vi "BarcodeScannerCodeforVideo.vi"() -> ()   [LabVIEW 2016]
uses:
  <vilib>/NXT/Block Support/NXT_InputPort.ctl
  <vilib>/NXT/Block Support/NXT_OutputPort.ctl
  <vilib>/NXT/Dual Mode Library/Sensors/Touch_Count.vi
  <vilib>/NXT/NXTIO Xnodes/NXTIONodeSubVIs/NXTMotorRunDistance.vi
  <vilib>/NXT/Dual Mode Library/Sensors/EV3_Color_Reflect.vi
  <vilib>/NXT/NXTIO Xnodes/NXTIONodeSubVIs/NXTStopMotors.vi
  <vilib>/NXT/Dual Mode Library/Sensors/EV3_Touch_Reset.vi
  <vilib>/NXT/NXTIO Xnodes/AddressXNode/NXTIOAddress.xnode
  <vilib>/NXT/NXTIO Xnodes/NXTIOXNode/NXTIO.xnode
  <vilib>/NXT/Subs/LVHSConnector.ctl
  <vilib>/NXT/LegoClasses/BrickReference/BrickReference.lvclass
panel:
  out "Marble Type 2 Code":i32[](array[numeric])
  out "Marble Count 2 Code":i32[](array[numeric])
  out "Marble Type 4":string
  out "Type 1 count 4":string
  out "Type 2 Count 4":string
  out "Marble Type 4 Code":i32[](array[numeric])
  out "Marble Count 4 Code":i32[](array[numeric])
  out "Marble Type 3":string
  out "Type 2 Count 3":string
  out "Type 1 Count 3":string
  out "Marble Count 3":i32[](array[numeric])
  out "Marble Type 3":i32[](array[numeric])
  out "Marble Type 2":string
  out "Type 2 Count 2":string
  out "Type 1 Count 2":string
  out "Marble Type code":i32[](array[numeric])
  out "Marble Size code":i32[](array[numeric])
  out "Marble Type":string
  out "Type 2 Count":string
  out "Type 1 Count":string
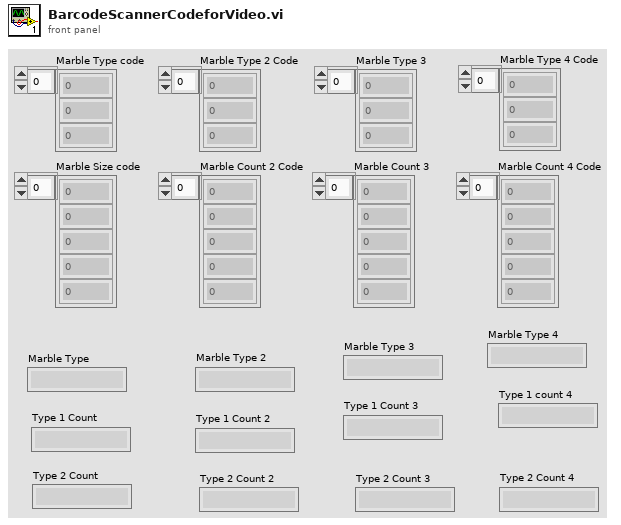
[diagram p1: front panel]
types:
  T1 = typedef "NXT_InputPort.ctl" = u32
  T2 = typedef "LVHSConnector.ctl" = refnum<class "BrickReference.lvclass">
  T3 = typedef "NXT_OutputPort.ctl" = u8
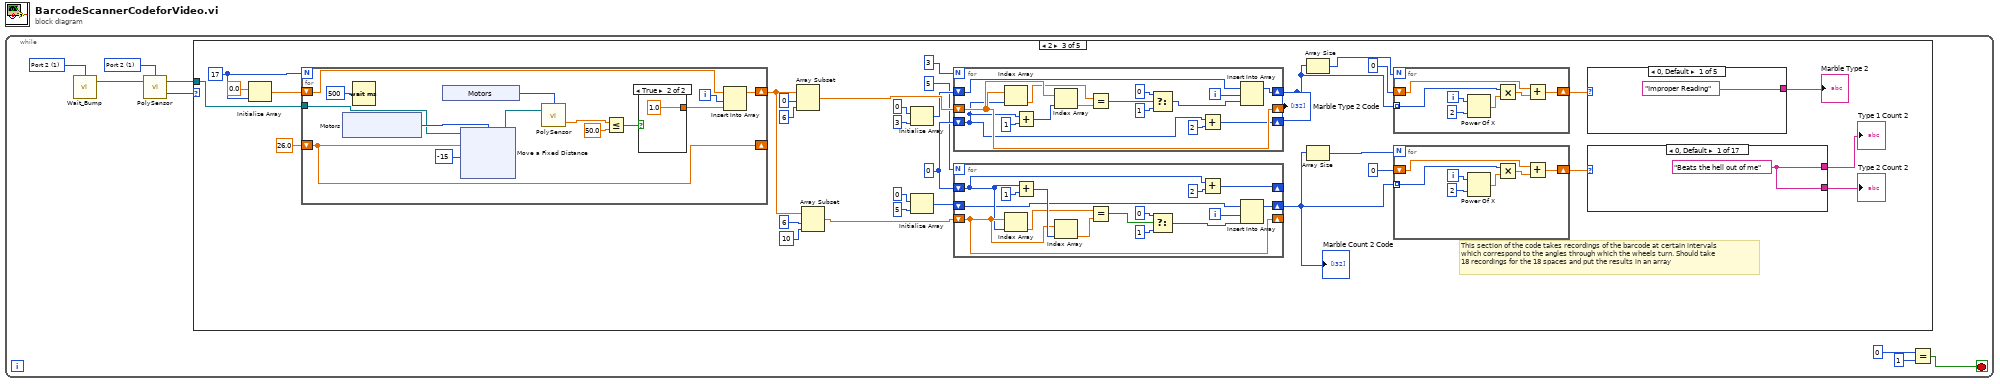
[diagram p0: block diagram]
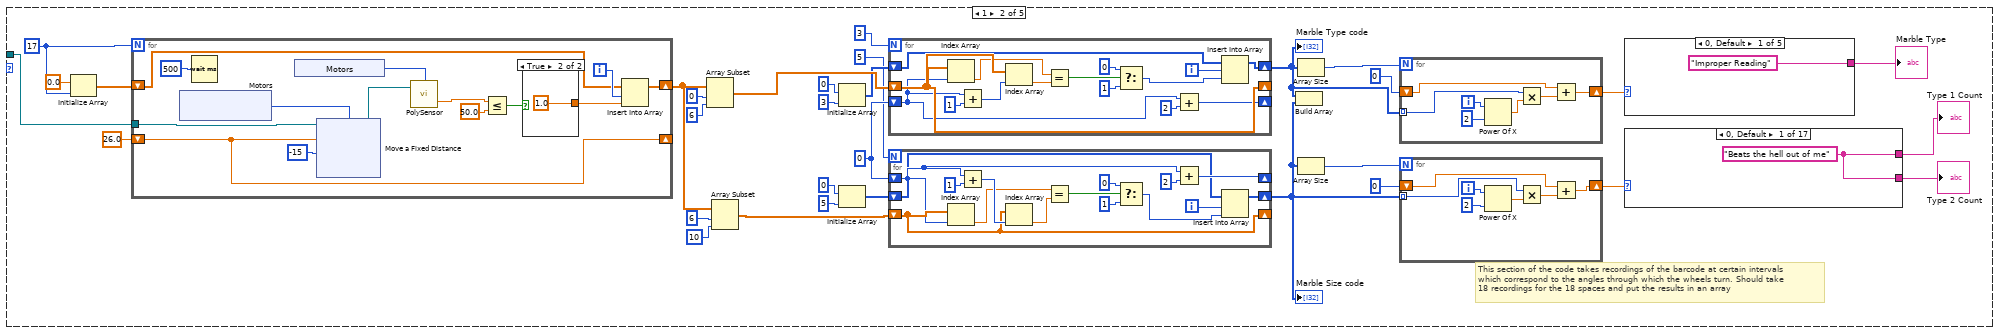
[diagram p3: hidden frame]
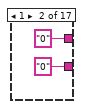
[diagram p4: hidden frame]
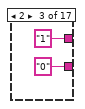
[diagram p5: hidden frame]
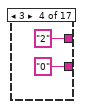
[diagram p6: hidden frame]
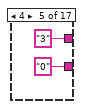
[diagram p7: hidden frame]
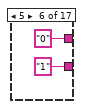
[diagram p8: hidden frame]
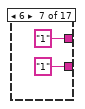
[diagram p9: hidden frame]
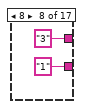
[diagram p10: hidden frame]
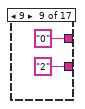
[diagram p11: hidden frame]
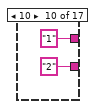
[diagram p12: hidden frame]
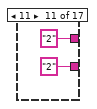
[diagram p13: hidden frame]
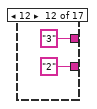
[diagram p14: hidden frame]
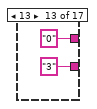
[diagram p15: hidden frame]
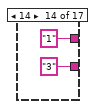
[diagram p16: hidden frame]
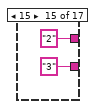
[diagram p17: hidden frame]
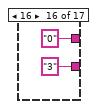
[diagram p18: hidden frame]
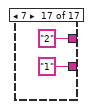
[diagram p19: hidden frame]
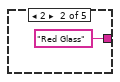
[diagram p20: hidden frame]
diagram:
  n1 = while {
    stop <- w1 stop-if-true
    w4 = T1 1 items=["Port 1", "Port 2", "Port 3", "Port 4"] ("Port (Port 1)")
    w5 = T1 1 items=["Port 1", "Port 2", "Port 3", "Port 4"] ("Port (Port 1)")
    n2 = call <vilib>:"Wait_Bump.vi"("Port (Port 1)"=w5) -> ("NXT/EV3"=w7:T2)  [unwired: 3 in]
    n3 = call-poly <vilib>:"PolySensor.vi"("NXT/EV3"=w7, "Port (Port 1)"=w4) -> ("Count"=w8:i16, "NXT/EV3"=w6:T2)  [unwired: 1 in]
    n4 = case shown="2" w8 {
      tunnel: w6 -> [_ w9 w151 w293 w444]
      frame 0, Default {
      }
      frame 1 {
        w23 = 0
        w40 = 17
        # "This section of the code takes recordings of the barcode at certain intervals\nwhich correspond to the angles through which the wheels turn. Should take\n18 recordings for the 18 spaces and put the results in an array"
        n5 = Initialize Array(0.0, w40) -> (w38:dbl[])
        n6 = for {
          N: w40 -> [_]
          shift-right: [w131] -> w15
          shift-left: w38 -> [w135]
          shift-right: [w128] -> _
          shift-left: 26.0 -> [w128]
          tunnel: w9 -> [w123]
          i -> [w136]
          n7 = xnode "Motors"() -> ("Motor"=w126:T3)
          n8 = Wait (ms)(milliseconds to wait=500) -> ()  [unwired: 1 out]
          n9 = xnode "Motors"() -> ("Sensor"=w130:T1)
          n10 = xnode "Move a Fixed Distance"("Speed 1"=i8 -15, "Distance 1"=w128, "Motors"=w126, "NXT/EV3"=w123) -> ("NXT/EV3"=w127:T2)
          n11 = call-poly <vilib>:"PolySensor.vi"("NXT/EV3"=w127, "Port (Port 1)"=w130) -> ("Scaled Value"=w129:sgl)  [unwired: 1 in, 1 out]
          n12 = Less Or Equal?(x=w129, y=50.0) -> (x <= y?=w133:bool)
          n13 = case shown="True" w133 {
            tunnel: [0.0 1.0] -> w132
            frame False {
            }
            frame True {
            }
          }
          n14 = Insert Into Array(array=w135, index=w136, new element=w132) -> (w131:dbl[])
        }
        n15 = Array Subset(array=w15, index=0, length=6) -> (w31:dbl[])
        n16 = Array Subset(array=w15, index=6, length=10) -> (w27:dbl[])
        n17 = Initialize Array(0, 3 ("dimension size")) -> (w29:i32[])
        n18 = Initialize Array(0, 5 ("dimension size")) -> (w24:i32[])
        n19 = for {
          N: 3 -> [_]
          shift-right: [w120] -> _
          shift-left: w31 -> [w120]
          shift-right: [w112] -> _
          shift-left: w23 -> [w113]
          shift-right: [w110] -> w14
          shift-left: w29 -> [w109]
          i -> [w108]
          n20 = Index Array(array=w120, index=w113) -> (element=w117:dbl)
          n21 = Add(x=w113, y=1) -> (x+y=w121:i32)
          n22 = Index Array(array=w120, index=w121) -> (element=w116:dbl)
          n23 = Equal?(x=w117, y=w116) -> (x = y?=w115:bool)
          n24 = Select(t=0, s=w115, f=1) -> (s? t:f=w114:i32)
          n25 = Add(x=w113, y=2) -> (x+y=w112:i32)
          n26 = Insert Into Array(array=w109, index=w108, new element=w114) -> (w110:i32[])
        }
        "Marble Type code" <- w14
        n27 = for {
          N: 5 -> [_]
          shift-right: [w105] -> _
          shift-left: w27 -> [w105]
          shift-right: [w97] -> _
          shift-left: w23 -> [w98]
          shift-right: [w95] -> w13
          shift-left: w24 -> [w94]
          i -> [w93]
          n28 = Index Array(array=w105, index=w98) -> (element=w102:dbl)
          n29 = Add(x=w98, y=1) -> (x+y=w106:i32)
          n30 = Index Array(array=w105, index=w106) -> (element=w101:dbl)
          n31 = Equal?(x=w102, y=w101) -> (x = y?=w100:bool)
          n32 = Select(t=0, s=w100, f=1) -> (s? t:f=w99:i32)
          n33 = Add(x=w98, y=2) -> (x+y=w97:i32)
          n34 = Insert Into Array(array=w94, index=w93, new element=w99) -> (w95:i32[])
        }
        "Marble Size code" <- w13
        n35 = Build Array(w14, w13) -> ()  [unwired: 1 out]
        n36 = Array Size(array=w14) -> (size(s)=w21:i32)
        n37 = Array Size(array=w13) -> (size(s)=w18:i32)
        n38 = for {
          N: w21 -> [_]
          tunnel: w14 -> [w51] mode=indexing
          shift-right: [w48] -> w19
          shift-left: 0 -> [w49]
          i -> [w53]
          n39 = Power Of X(1:2, 2:w53) -> (0:w52:dbl)
          n40 = Multiply(x=w51, y=w52) -> (x*y=w50:dbl)
          n41 = Add(x=w49, y=w50) -> (x+y=w48:dbl)
        }
        n42 = for {
          N: w18 -> [_]
          tunnel: w13 -> [w44] mode=indexing
          shift-right: [w41] -> w16
          shift-left: 0 -> [w42]
          i -> [w46]
          n43 = Power Of X(1:2, 2:w46) -> (0:w45:dbl)
          n44 = Multiply(x=w44, y=w45) -> (x*y=w43:dbl)
          n45 = Add(x=w42, y=w43) -> (x+y=w41:dbl)
        }
        n46 = case shown="0, Default" w19 {
          tunnel: ["Improper Reading" "Red Glass" "Blue Glass" "White Glass" "Steel/HDPE"] -> w10
          frame 0, Default {
          }
          frame 2 {
          }
          frame 3 {
          }
          frame 1 {
          }
          frame 4 {
          }
        }
        "Marble Type" <- w10
        n47 = case shown="0, Default" w16 {
          tunnel: [w55 "0" "1" "2" "3" "0" "1" "3" "0" "1" "2" "3" "0" "1" "2" "0" "2"] -> w12
          tunnel: [w55 "0" "0" "0" "0" "1" "1" "1" "2" "2" "2" "2" "3" "3" "3" "3" "1"] -> w11
          frame 0, Default {
            w55 = "Beats the hell out of me"
          }
          frame 1 {
          }
          frame 2 {
          }
          frame 3 {
          }
          frame 4 {
          }
          frame 5 {
          }
          frame 6 {
          }
          frame 8 {
          }
          frame 9 {
          }
          frame 10 {
          }
          frame 11 {
          }
          frame 12 {
          }
          frame 13 {
          }
          frame 14 {
          }
          frame 15 {
          }
          frame 16 {
          }
          frame 7 {
          }
        }
        "Type 2 Count" <- w11
        "Type 1 Count" <- w12
      }
      frame 2 {
        w165 = 0
        w182 = 17
        # "This section of the code takes recordings of the barcode at certain intervals\nwhich correspond to the angles through which the wheels turn. Should take\n18 recordings for the 18 spaces and put the results in an array"
        n48 = Initialize Array(0.0, w182) -> (w180:dbl[])
        n49 = for {
          N: w182 -> [_]
          shift-right: [w273] -> w154
          shift-left: w180 -> [w277]
          shift-right: [w270] -> _
          shift-left: 26.0 -> [w270]
          tunnel: w151 -> [w265]
          i -> [w278]
          n50 = xnode "Motors"() -> ("Motor"=w268:T3)
          n51 = Wait (ms)(milliseconds to wait=500) -> ()  [unwired: 1 out]
          n52 = xnode "Motors"() -> ("Sensor"=w272:T1)
          n53 = xnode "Move a Fixed Distance"("Speed 1"=i8 -15, "Distance 1"=w270, "Motors"=w268, "NXT/EV3"=w265) -> ("NXT/EV3"=w269:T2)
          n54 = call-poly <vilib>:"PolySensor.vi"("NXT/EV3"=w269, "Port (Port 1)"=w272) -> ("Scaled Value"=w271:sgl)  [unwired: 1 in, 1 out]
          n55 = Less Or Equal?(x=w271, y=50.0) -> (x <= y?=w275:bool)
          n56 = case shown="True" w275 {
            tunnel: [0.0 1.0] -> w274
            frame False {
            }
            frame True {
            }
          }
          n57 = Insert Into Array(array=w277, index=w278, new element=w274) -> (w273:dbl[])
        }
        n58 = Array Subset(array=w154, index=0, length=6) -> (w173:dbl[])
        n59 = Array Subset(array=w154, index=6, length=10) -> (w169:dbl[])
        n60 = Initialize Array(0, 3 ("dimension size")) -> (w171:i32[])
        n61 = Initialize Array(0, 5 ("dimension size")) -> (w166:i32[])
        n62 = for {
          N: 3 -> [_]
          shift-right: [w262] -> _
          shift-left: w173 -> [w262]
          shift-right: [w254] -> _
          shift-left: w165 -> [w255]
          shift-right: [w252] -> w153
          shift-left: w171 -> [w251]
          i -> [w250]
          n63 = Index Array(array=w262, index=w255) -> (element=w259:dbl)
          n64 = Add(x=w255, y=1) -> (x+y=w263:i32)
          n65 = Index Array(array=w262, index=w263) -> (element=w258:dbl)
          n66 = Equal?(x=w259, y=w258) -> (x = y?=w257:bool)
          n67 = Select(t=0, s=w257, f=1) -> (s? t:f=w256:i32)
          n68 = Add(x=w255, y=2) -> (x+y=w254:i32)
          n69 = Insert Into Array(array=w251, index=w250, new element=w256) -> (w252:i32[])
        }
        "Marble Type 2 Code" <- w153
        n70 = for {
          N: 5 -> [_]
          shift-right: [w247] -> _
          shift-left: w169 -> [w247]
          shift-right: [w239] -> _
          shift-left: w165 -> [w240]
          shift-right: [w237] -> w152
          shift-left: w166 -> [w236]
          i -> [w235]
          n71 = Index Array(array=w247, index=w240) -> (element=w244:dbl)
          n72 = Add(x=w240, y=1) -> (x+y=w248:i32)
          n73 = Index Array(array=w247, index=w248) -> (element=w243:dbl)
          n74 = Equal?(x=w244, y=w243) -> (x = y?=w242:bool)
          n75 = Select(t=0, s=w242, f=1) -> (s? t:f=w241:i32)
          n76 = Add(x=w240, y=2) -> (x+y=w239:i32)
          n77 = Insert Into Array(array=w236, index=w235, new element=w241) -> (w237:i32[])
        }
        "Marble Count 2 Code" <- w152
        n78 = Array Size(array=w153) -> (size(s)=w160:i32)
        n79 = Array Size(array=w152) -> (size(s)=w157:i32)
        n80 = for {
          N: w160 -> [_]
          tunnel: w153 -> [w193] mode=indexing
          shift-right: [w190] -> w158
          shift-left: 0 -> [w191]
          i -> [w195]
          n81 = Power Of X(1:2, 2:w195) -> (0:w194:dbl)
          n82 = Multiply(x=w193, y=w194) -> (x*y=w192:dbl)
          n83 = Add(x=w191, y=w192) -> (x+y=w190:dbl)
        }
        n84 = for {
          N: w157 -> [_]
          tunnel: w152 -> [w186] mode=indexing
          shift-right: [w183] -> w155
          shift-left: 0 -> [w184]
          i -> [w188]
          n85 = Power Of X(1:2, 2:w188) -> (0:w187:dbl)
          n86 = Multiply(x=w186, y=w187) -> (x*y=w185:dbl)
          n87 = Add(x=w184, y=w185) -> (x+y=w183:dbl)
        }
        n88 = case shown="0, Default" w158 {
          tunnel: ["Improper Reading" "Red Glass" "Blue Glass" "White Glass" "Steel/HDPE"] -> w163
          frame 0, Default {
          }
          frame 2 {
          }
          frame 3 {
          }
          frame 1 {
          }
          frame 4 {
          }
        }
        "Marble Type 2" <- w163
        n89 = case shown="0, Default" w155 {
          tunnel: [w197 "0" "1" "2" "3" "0" "1" "3" "0" "1" "2" "3" "0" "1" "2" "0" "2"] -> w161
          tunnel: [w197 "0" "0" "0" "0" "1" "1" "1" "2" "2" "2" "2" "3" "3" "3" "3" "1"] -> w162
          frame 0, Default {
            w197 = "Beats the hell out of me"
          }
          frame 1 {
          }
          frame 2 {
          }
          frame 3 {
          }
          frame 4 {
          }
          frame 5 {
          }
          frame 6 {
          }
          frame 8 {
          }
          frame 9 {
          }
          frame 10 {
          }
          frame 11 {
          }
          frame 12 {
          }
          frame 13 {
          }
          frame 14 {
          }
          frame 15 {
          }
          frame 16 {
          }
          frame 7 {
          }
        }
        "Type 2 Count 2" <- w162
        "Type 1 Count 2" <- w161
      }
      frame 3 {
        w315 = 0
        w298 = 17
        # "This section of the code takes recordings of the barcode at certain intervals\nwhich correspond to the angles through which the wheels turn. Should take\n18 recordings for the 18 spaces and put the results in an array"
        n90 = Initialize Array(0.0, w298) -> (w300:dbl[])
        n91 = for {
          N: w298 -> [_]
          shift-right: [w416] -> w323
          shift-left: w300 -> [w420]
          shift-right: [w413] -> _
          shift-left: 26.0 -> [w413]
          tunnel: w293 -> [w407]
          i -> [w421]
          n92 = xnode "Motors"() -> ("Motor"=w408:T3)
          n93 = xnode "Motors"() -> ("Motor"=w411:T3)
          n94 = Wait (ms)(milliseconds to wait=500) -> ()  [unwired: 1 out]
          n95 = xnode "Stop Motors"("Motors"=w408) -> ()  [unwired: 1 in, 1 out]
          n96 = xnode "Motors"() -> ("Sensor"=w415:T1)
          n97 = xnode "Move a Fixed Distance"("Speed 1"=i8 -15, "Distance 1"=w413, "Motors"=w411, "NXT/EV3"=w407) -> ("NXT/EV3"=w412:T2)
          n98 = call-poly <vilib>:"PolySensor.vi"("NXT/EV3"=w412, "Port (Port 1)"=w415) -> ("Scaled Value"=w414:sgl)  [unwired: 1 in, 1 out]
          n99 = Less Or Equal?(x=w414, y=50.0) -> (x <= y?=w418:bool)
          n100 = case shown="True" w418 {
            tunnel: [0.0 1.0] -> w417
            frame False {
            }
            frame True {
            }
          }
          n101 = Insert Into Array(array=w420, index=w421, new element=w417) -> (w416:dbl[])
        }
        n102 = Array Subset(array=w323, index=0, length=6) -> (w307:dbl[])
        n103 = Array Subset(array=w323, index=6, length=10) -> (w311:dbl[])
        n104 = Initialize Array(0, 3 ("dimension size")) -> (w309:i32[])
        n105 = for {
          N: 3 -> [_]
          shift-right: [w404] -> _
          shift-left: w307 -> [w404]
          shift-right: [w396] -> _
          shift-left: w315 -> [w397]
          shift-right: [w394] -> w324
          shift-left: w309 -> [w393]
          i -> [w392]
          n106 = Index Array(array=w404, index=w397) -> (element=w401:dbl)
          n107 = Add(x=w397, y=1) -> (x+y=w405:i32)
          n108 = Index Array(array=w404, index=w405) -> (element=w400:dbl)
          n109 = Equal?(x=w401, y=w400) -> (x = y?=w399:bool)
          n110 = Select(t=0, s=w399, f=1) -> (s? t:f=w398:i32)
          n111 = Add(x=w397, y=2) -> (x+y=w396:i32)
          n112 = Insert Into Array(array=w393, index=w392, new element=w398) -> (w394:i32[])
        }
        "Marble Type 3" <- w324
        n113 = Initialize Array(0, 5 ("dimension size")) -> (w314:i32[])
        n114 = for {
          N: 5 -> [_]
          shift-right: [w389] -> _
          shift-left: w311 -> [w389]
          shift-right: [w381] -> _
          shift-left: w315 -> [w382]
          shift-right: [w379] -> w294
          shift-left: w314 -> [w378]
          i -> [w377]
          n115 = Index Array(array=w389, index=w382) -> (element=w386:dbl)
          n116 = Add(x=w382, y=1) -> (x+y=w390:i32)
          n117 = Index Array(array=w389, index=w390) -> (element=w385:dbl)
          n118 = Equal?(x=w386, y=w385) -> (x = y?=w384:bool)
          n119 = Select(t=0, s=w384, f=1) -> (s? t:f=w383:i32)
          n120 = Add(x=w382, y=2) -> (x+y=w381:i32)
          n121 = Insert Into Array(array=w378, index=w377, new element=w383) -> (w379:i32[])
        }
        "Marble Count 3" <- w294
        n122 = Array Size(array=w324) -> (size(s)=w317:i32)
        n123 = Array Size(array=w294) -> (size(s)=w320:i32)
        n124 = for {
          N: w317 -> [_]
          tunnel: w324 -> [w335] mode=indexing
          shift-right: [w332] -> w319
          shift-left: 0 -> [w333]
          i -> [w337]
          n125 = Power Of X(1:2, 2:w337) -> (0:w336:dbl)
          n126 = Multiply(x=w335, y=w336) -> (x*y=w334:dbl)
          n127 = Add(x=w333, y=w334) -> (x+y=w332:dbl)
        }
        n128 = for {
          N: w320 -> [_]
          tunnel: w294 -> [w328] mode=indexing
          shift-right: [w325] -> w322
          shift-left: 0 -> [w326]
          i -> [w330]
          n129 = Power Of X(1:2, 2:w330) -> (0:w329:dbl)
          n130 = Multiply(x=w328, y=w329) -> (x*y=w327:dbl)
          n131 = Add(x=w326, y=w327) -> (x+y=w325:dbl)
        }
        n132 = case shown="0, Default" w319 {
          tunnel: ["Improper Reading" "Red Glass" "Blue Glass" "White Glass" "Steel/HDPE"] -> w295
          frame 0, Default {
          }
          frame 2 {
          }
          frame 3 {
          }
          frame 1 {
          }
          frame 4 {
          }
        }
        "Marble Type 3" <- w295
        n133 = case shown="0, Default" w322 {
          tunnel: [w339 "0" "1" "2" "3" "0" "1" "3" "0" "1" "2" "3" "0" "1" "2" "0" "2"] -> w297
          tunnel: [w339 "0" "0" "0" "0" "1" "1" "1" "2" "2" "2" "2" "3" "3" "3" "3" "1"] -> w296
          frame 0, Default {
            w339 = "Beats the hell out of me"
          }
          frame 1 {
          }
          frame 2 {
          }
          frame 3 {
          }
          frame 4 {
          }
          frame 5 {
          }
          frame 6 {
          }
          frame 8 {
          }
          frame 9 {
          }
          frame 10 {
          }
          frame 11 {
          }
          frame 12 {
          }
          frame 13 {
          }
          frame 14 {
          }
          frame 15 {
          }
          frame 16 {
          }
          frame 7 {
          }
        }
        "Type 2 Count 3" <- w296
        "Type 1 Count 3" <- w297
      }
      frame 4 {
        w443 = T1 1 items=["Port 1", "Port 2", "Port 3", "Port 4"] ("Port (Port 1)")
        w465 = 0
        w448 = 17
        # "This section of the code takes recordings of the barcode at certain intervals\nwhich correspond to the angles through which the wheels turn. Should take\n18 recordings for the 18 spaces and put the results in an array"
        n134 = Initialize Array(0.0, w448) -> (w450:dbl[])
        n135 = for {
          N: w448 -> [_]
          shift-right: [w569] -> w473
          shift-left: w450 -> [w573]
          shift-right: [w566] -> _
          shift-left: 26.0 -> [w566]
          tunnel: w444 -> [w560]
          tunnel: [w558] -> w442
          i -> [w574]
          n136 = xnode "Motors"() -> ("Motor"=w564:T3)
          n137 = Wait (ms)(milliseconds to wait=500) -> ()  [unwired: 1 out]
          n138 = xnode "Motors"() -> ("Sensor"=w568:T1)
          n139 = xnode "Move a Fixed Distance"("Speed 1"=i8 -15, "Distance 1"=w566, "Motors"=w564, "NXT/EV3"=w560) -> ("NXT/EV3"=w565:T2)
          n140 = xnode "Motors"() -> ("Motor"=w561:T3)
          n141 = call-poly <vilib>:"PolySensor.vi"("NXT/EV3"=w565, "Port (Port 1)"=w568) -> ("Scaled Value"=w567:sgl, "NXT/EV3"=w559:T2)  [unwired: 1 in]
          n142 = xnode "Stop Motors"("Motors"=w561, "NXT/EV3"=w559) -> ("NXT/EV3"=w558:T2)
          n143 = Less Or Equal?(x=w567, y=50.0) -> (x <= y?=w571:bool)
          n144 = case shown="True" w571 {
            tunnel: [0.0 1.0] -> w570
            frame False {
            }
            frame True {
            }
          }
          n145 = Insert Into Array(array=w573, index=w574, new element=w570) -> (w569:dbl[])
        }
        n146 = Array Subset(array=w473, index=0, length=6) -> (w457:dbl[])
        n147 = Array Subset(array=w473, index=6, length=10) -> (w461:dbl[])
        n148 = call-poly <vilib>:"PolySensor.vi"("NXT/EV3"=w442, "Port (Port 1)"=w443) -> ()  [unwired: 2 in, 1 out]
        n149 = Initialize Array(0, 3 ("dimension size")) -> (w459:i32[])
        n150 = for {
          N: 3 -> [_]
          shift-right: [w555] -> _
          shift-left: w457 -> [w555]
          shift-right: [w547] -> _
          shift-left: w465 -> [w548]
          shift-right: [w545] -> w474
          shift-left: w459 -> [w544]
          i -> [w543]
          n151 = Index Array(array=w555, index=w548) -> (element=w552:dbl)
          n152 = Add(x=w548, y=1) -> (x+y=w556:i32)
          n153 = Index Array(array=w555, index=w556) -> (element=w551:dbl)
          n154 = Equal?(x=w552, y=w551) -> (x = y?=w550:bool)
          n155 = Select(t=0, s=w550, f=1) -> (s? t:f=w549:i32)
          n156 = Add(x=w548, y=2) -> (x+y=w547:i32)
          n157 = Insert Into Array(array=w544, index=w543, new element=w549) -> (w545:i32[])
        }
        "Marble Type 4 Code" <- w474
        n158 = Initialize Array(0, 5 ("dimension size")) -> (w464:i32[])
        n159 = for {
          N: 5 -> [_]
          shift-right: [w540] -> _
          shift-left: w461 -> [w540]
          shift-right: [w532] -> _
          shift-left: w465 -> [w533]
          shift-right: [w530] -> w475
          shift-left: w464 -> [w529]
          i -> [w528]
          n160 = Index Array(array=w540, index=w533) -> (element=w537:dbl)
          n161 = Add(x=w533, y=1) -> (x+y=w541:i32)
          n162 = Index Array(array=w540, index=w541) -> (element=w536:dbl)
          n163 = Equal?(x=w537, y=w536) -> (x = y?=w535:bool)
          n164 = Select(t=0, s=w535, f=1) -> (s? t:f=w534:i32)
          n165 = Add(x=w533, y=2) -> (x+y=w532:i32)
          n166 = Insert Into Array(array=w529, index=w528, new element=w534) -> (w530:i32[])
        }
        "Marble Count 4 Code" <- w475
        n167 = Array Size(array=w474) -> (size(s)=w467:i32)
        n168 = Array Size(array=w475) -> (size(s)=w470:i32)
        n169 = for {
          N: w467 -> [_]
          tunnel: w474 -> [w486] mode=indexing
          shift-right: [w483] -> w469
          shift-left: 0 -> [w484]
          i -> [w488]
          n170 = Power Of X(1:2, 2:w488) -> (0:w487:dbl)
          n171 = Multiply(x=w486, y=w487) -> (x*y=w485:dbl)
          n172 = Add(x=w484, y=w485) -> (x+y=w483:dbl)
        }
        n173 = for {
          N: w470 -> [_]
          tunnel: w475 -> [w479] mode=indexing
          shift-right: [w476] -> w472
          shift-left: 0 -> [w477]
          i -> [w481]
          n174 = Power Of X(1:2, 2:w481) -> (0:w480:dbl)
          n175 = Multiply(x=w479, y=w480) -> (x*y=w478:dbl)
          n176 = Add(x=w477, y=w478) -> (x+y=w476:dbl)
        }
        n177 = case shown="2" w469 {
          tunnel: ["Improper Reading" "Red Glass" "Blue Glass" "White Glass" "Steel/HDPE"] -> w447
          frame 0, Default {
          }
          frame 2 {
          }
          frame 3 {
          }
          frame 1 {
          }
          frame 4 {
          }
        }
        "Marble Type 4" <- w447
        n178 = case shown="3" w472 {
          tunnel: [w490 "0" "1" "2" "3" "0" "1" "3" "0" "1" "2" "3" "0" "1" "2" "0" "2"] -> w446
          tunnel: [w490 "0" "0" "0" "0" "1" "1" "1" "2" "2" "2" "2" "3" "3" "3" "3" "1"] -> w445
          frame 0, Default {
            w490 = "Beats the hell out of me"
          }
          frame 1 {
          }
          frame 2 {
          }
          frame 3 {
          }
          frame 4 {
          }
          frame 5 {
          }
          frame 6 {
          }
          frame 8 {
          }
          frame 9 {
          }
          frame 10 {
          }
          frame 11 {
          }
          frame 12 {
          }
          frame 13 {
          }
          frame 14 {
          }
          frame 15 {
          }
          frame 16 {
          }
          frame 7 {
          }
        }
        "Type 1 count 4" <- w445
        "Type 2 Count 4" <- w446
      }
    }
    n179 = Equal?(x=0, y=1) -> (x = y?=w1:bool)
  }
